vi "Main_VI.vi"() -> ()   [LabVIEW 2023]
uses:
  TypeDef/State.ctl
  TypeDef/Data_Cluster.ctl
  TypeDef/Units.ctl
  TypeDef/Method_Info.ctl
  TypeDef/Method_Types.ctl
panel:
  out "Cluster of Units 2":T1
  out "dmin":dbl format="%#_7g"
  out "dmax":dbl format="%#_7g"
  out "Fundamental Deviation":dbl format="%#_7g"
  out "Cluster of Units":T2
  out "Dmin":dbl format="%#_7g"
  out "Dmax":dbl
  out "Tolerance Grade (IT)":dbl format="%#_7g"
  in  "Help Button":bool
  in  "Close Button":bool
  in  "Base Size":dbl
  in  "Units":T3
  out "Method_Description":string
  out "Symbol":string
  in  "Method_Fit":T4
  in  "error in":errorcluster
  # "Shaft"
  # "Hole"
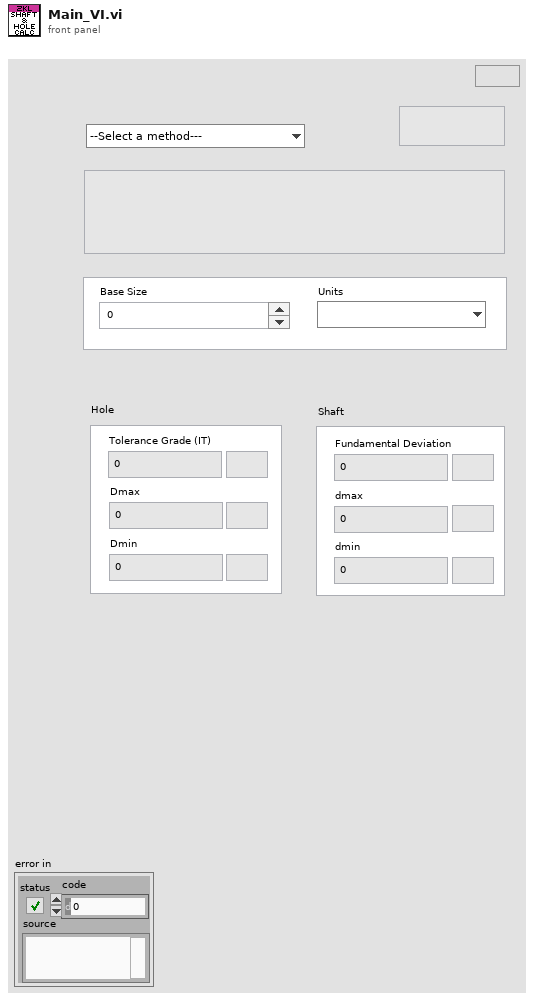
[diagram p1: front panel]
types:
  T1 = cluster{"Units_FundamentalDev":string, "Units_dmax":string, "Units_dmin":string}
  T2 = cluster{"units_it":string, "units_Dmax\nUnits_Dmax":string, "Units_Dmin":string}
  T3 = typedef "Units.ctl" = enum16{"", "mm", "in"}
  T4 = typedef "Method_Types.ctl" = enum16{"--Select a method---", "Clearance (Loose Running Fit)", "Clearance (Free Running Fit)", "Clearance (Close Running Fit)", "Clearance (Sliding Fit)", "Clearance (Locational Fit)", "Transition (Locational A)", "Transition (Locational B)", "Interference (Locational Fit)", "Interference (Force Fit)", "Interference (Medium Drive Fit)"}
  T5 = typedef "Method_Info.ctl" = cluster{"Method":string, "Sym":string, "Tolerance Grade Number":i32, "Shaft":i32, "Group":string}
  T6 = typedef "State.ctl" = enum16{"Wait for something", "Method_Description", "Tolerance Grade Hole", "Dmax-min", "Shaft Fudamental", "Shaft Tolerance Grade", "dmax-dmin", "Write Unit", "End"}
  T7 = typedef "Data_Cluster.ctl" = cluster{"Basic Size ":dbl, "Unit":T3, "Data":T5, "Tolerance Grade Hole  ":dbl, "Fundamental":dbl, "Tables Main Path":path, "Tolerance Grade Shaft":dbl}
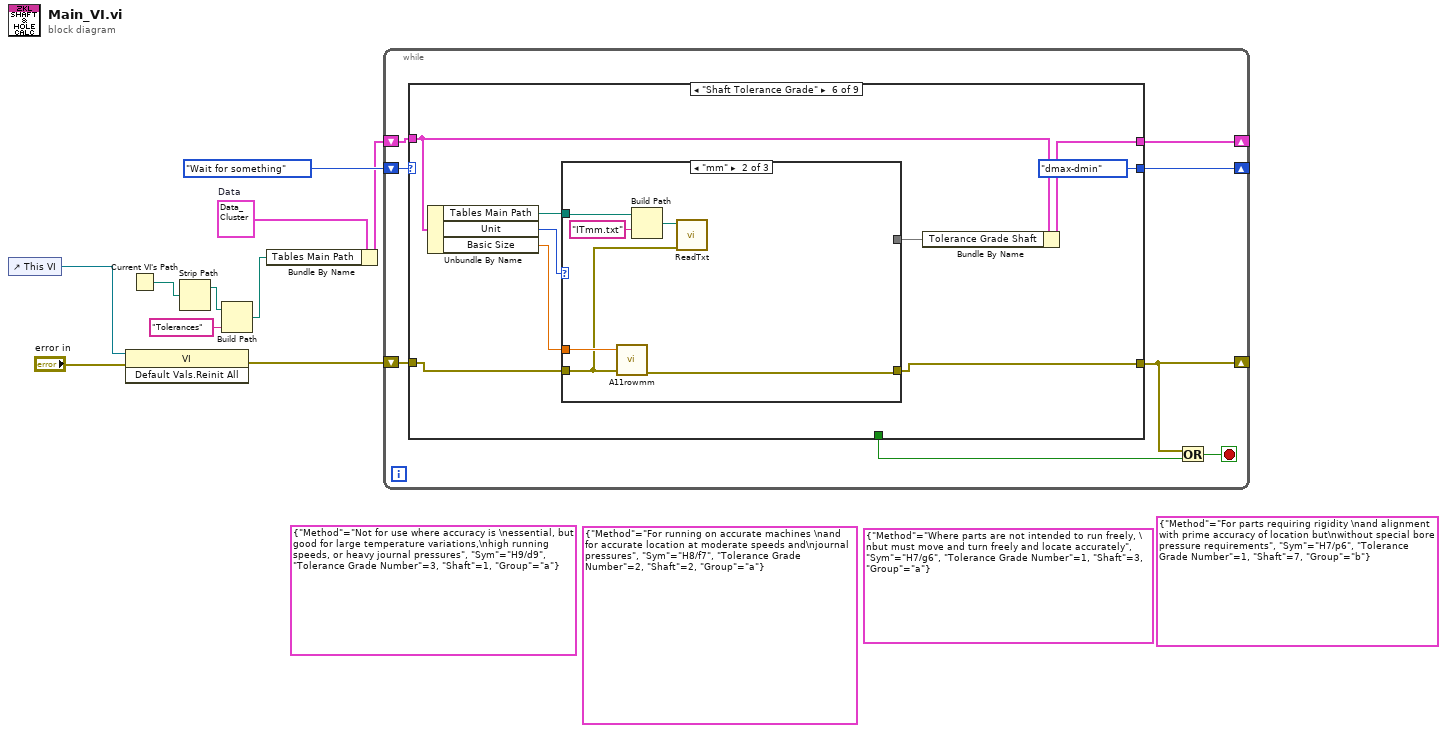
[diagram p0: block diagram]
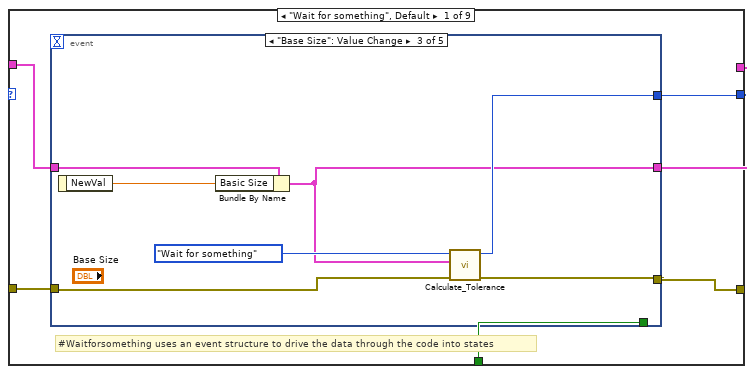
[diagram p2: hidden frame]
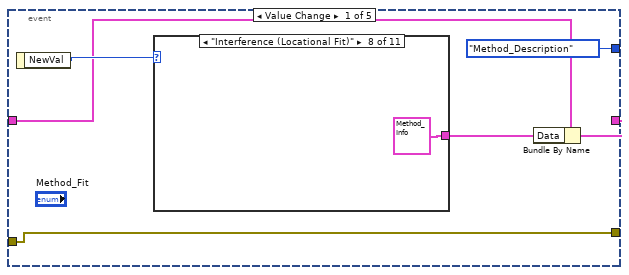
[diagram p3: hidden frame]
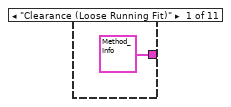
[diagram p4: hidden frame]
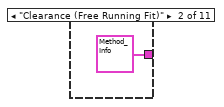
[diagram p5: hidden frame]
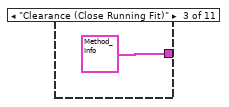
[diagram p6: hidden frame]
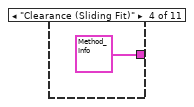
[diagram p7: hidden frame]
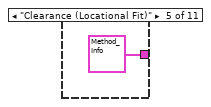
[diagram p8: hidden frame]
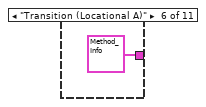
[diagram p9: hidden frame]
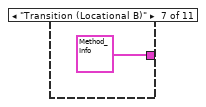
[diagram p10: hidden frame]
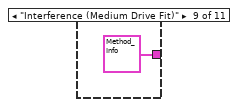
[diagram p11: hidden frame]
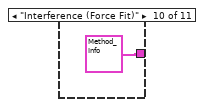
[diagram p12: hidden frame]
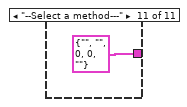
[diagram p13: hidden frame]
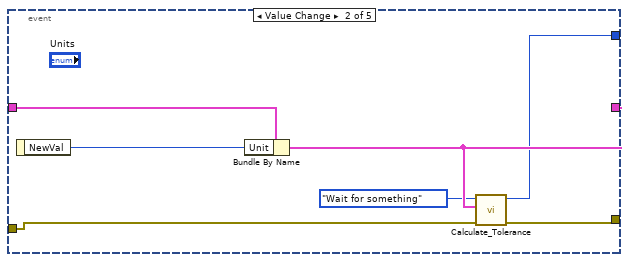
[diagram p14: hidden frame]
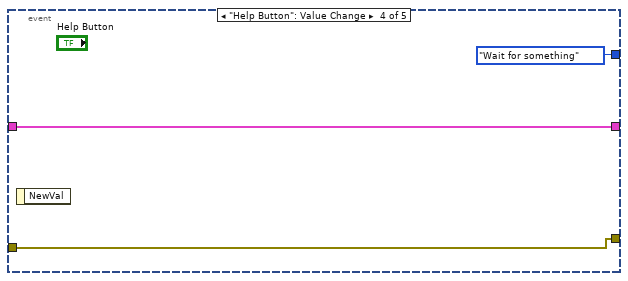
[diagram p15: hidden frame]
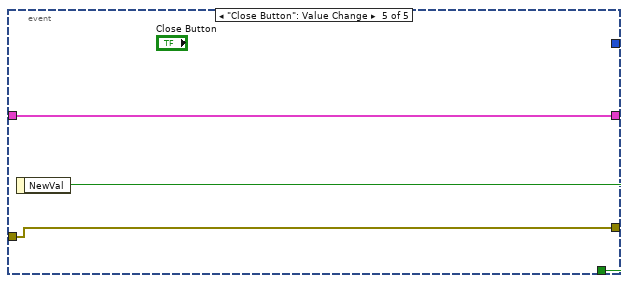
[diagram p16: hidden frame]
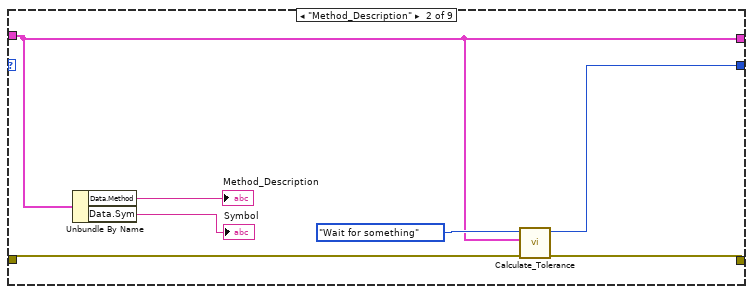
[diagram p17: hidden frame]
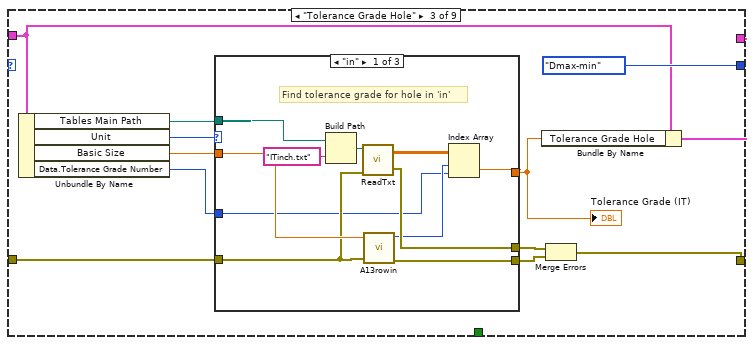
[diagram p18: hidden frame]
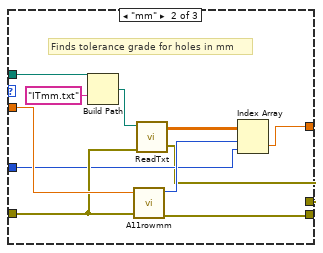
[diagram p19: hidden frame]
diagram:
  (unwired) T5 {"Method"="For parts requiring rigidity \nand alignment with prime accuracy of location but\nwithout special bore pressure requirements", "Sym"="H7/p6", "Tolerance Grade Number"=1, "Shaft"=7, "Group"="b"}
  (unwired) T5 {"Method"="Where parts are not intended to run freely, \nbut must move and turn freely and locate accurately", "Sym"="H7/g6", "Tolerance Grade Number"=1, "Shaft"=3, "Group"="a"}
  (unwired) T5 {"Method"="For running on accurate machines \nand for accurate location at moderate speeds and\njournal pressures", "Sym"="H8/f7", "Tolerance Grade Number"=2, "Shaft"=2, "Group"="a"}
  (unwired) T5 {"Method"="Not for use where accuracy is \nessential, but good for large temperature variations,\nhigh running speeds, or heavy journal pressures", "Sym"="H9/d9", "Tolerance Grade Number"=3, "Shaft"=1, "Group"="a"}
  w10 = T7 {"Basic Size "=0.0, "Unit"=enum."", "Data"={"Method"="", "Sym"="", "Tolerance Grade Number"=0, "Shaft"=0, "Group"=""}, "Tolerance Grade Hole  "=0.0, "Fundamental"=0.0, "Tables Main Path"=path "", "Tolerance Grade Shaft"=0.0}  # Data
  n1 = control-ref of="This VI"() -> (w8:refnum<vi>)
  n2 = invoke class="VI" method="Default Vals.Reinit All"(reference=w8, error in="error in") -> (error out=w6:errorcluster)  [unwired: 1 in, 2 out]
  n3 = Current VI's Path() -> (path=w4:path)
  n4 = Strip Path(path=w4) -> (stripped path=w2:path)  [unwired: 1 out]
  n5 = Build Path(base path=w2, name or relative path="Tolerances") -> (appended path=w3:path)
  n6 = Bundle By Name(cluster=w10, "Tables Main Path"=w3) -> (w5:T7)
  n7 = while {
    shift-right: [w17] -> _
    shift-left: w5 -> [w18]
    shift-right: [w15] -> _
    shift-left: State."Wait for something" -> [w16]
    shift-right: [w11] -> _
    shift-left: w6 -> [w14]
    stop <- w13 stop-if-true
    n8 = case shown="\"Shaft Tolerance Grade\"" w16 {
      tunnel: [w21 w63 w77 w105 w122 w161 w182 w202 w213] -> w17
      tunnel: w18 -> [w24 w63 w76 w105 w131 w163 w182 w202 w213]
      tunnel: [w19 w62 State."Dmax-min" State."Shaft Fudamental" State."Shaft Tolerance Grade" State."dmax-dmin" State."Write Unit" State."Wait for something" State."Wait for something"] -> w15
      tunnel: [w20 w66 w69 w106 w126 w159 w184 w208 w212] -> w11
      tunnel: w14 -> [w23 w65 w79 w107 w128 w160 w184 w209 w212]
      tunnel: [w22 _ _ _ _ _ _ _ _] -> w12
      frame "Wait for something", Default {
        # "#Waitforsomething uses an event structure to drive the data through the code into states"
        n9 = event shown="[2] \"Base Size\": Value Change" {
          selector: _ -> [_ _ _ _ _]
          dyn-events: _ -> [_ _ _ _ _]
          timeout: _ -> [_ _ _ _ _]
          tunnel: [w26 w46 w49 w58 w61] -> w21
          tunnel: w24 -> [w29 w47 w55 w58 w61]
          tunnel: [State."Method_Description" w42 w51 State."Wait for something" _] -> w19
          tunnel: w23 -> [w28 w45 w52 w56 w59]
          tunnel: [_ _ _ _ w60] -> w22
          tunnel: [w28 w43 w53 w56 w59] -> w20
          event Value Change {
            n10 = event-data() -> ("NewVal"=w30:T4)  [unwired: 1 in]
            n11 = case shown="\"Interference (Locational Fit)\"" w30 {
              tunnel: [T5 {"Method"="For wide commercial tolerances or allowances on external members", "Sym"="H11/c11", "Tolerance Grade Number"=5, "Shaft"=0, "Group"="a"} T5 {"Method"="Not for use where accuracy is \nessential, but good for large temperature variations,\nhigh running speeds, or heavy journal pressures", "Sym"="H9/d9", "Tolerance Grade Number"=3, "Shaft"=1, "Group"="a"} T5 {"Method"="For running on accurate machines \nand for accurate location at moderate speeds and\njournal pressures", "Sym"="H8/f7", "Tolerance Grade Number"=2, "Shaft"=2, "Group"="a"} T5 {"Method"="Where parts are not intended to run freely, \nbut must move and turn freely and locate accurately", "Sym"="H7/g6", "Tolerance Grade Number"=1, "Shaft"=3, "Group"="a"} T5 {"Method"="Provides snug fit for location \nof stationary parts, but can be freely assembled and\ndisassembled", "Sym"="H7/h6", "Tolerance Grade Number"=1, "Shaft"=4, "Group"="a"} T5 {"Method"="For accurate location, a \ncompromise between clearance and interference", "Sym"="H7/k6", "Tolerance Grade Number"=1, "Shaft"=5, "Group"="b"} T5 {"Method"="For more accurate location \nwhere greater interference is permissible", "Sym"="H7/n6", "Tolerance Grade Number"=1, "Shaft"=6, "Group"="b"} T5 {"Method"="For parts requiring rigidity \nand alignment with prime accuracy of location but\nwithout special bore pressure requirements", "Sym"="H7/p6", "Tolerance Grade Number"=1, "Shaft"=7, "Group"="b"} T5 {"Method"="For ordinary steel parts or shrink fits on\nlight sections, the tightest fit usable with cast iron", "Sym"="H7/s6", "Tolerance Grade Number"=1, "Shaft"=8, "Group"="b"} T5 {"Method"="Suitable for parts that can be highly stressed \nor for shrink fits where the heavy pressing forces required\nare impractical", "Sym"="H7/u6", "Tolerance Grade Number"=1, "Shaft"=9, "Group"="b"} T5 {"Method"="", "Sym"="", "Tolerance Grade Number"=0, "Shaft"=0, "Group"=""}] -> w25
              frame "Clearance (Loose Running Fit)" {
              }
              frame "Clearance (Free Running Fit)" {
              }
              frame "Clearance (Close Running Fit)" {
              }
              frame "Clearance (Sliding Fit)" {
              }
              frame "Clearance (Locational Fit)" {
              }
              frame "Transition (Locational A)" {
              }
              frame "Transition (Locational B)" {
              }
              frame "Interference (Locational Fit)" {
              }
              frame "Interference (Medium Drive Fit)" {
              }
              frame "Interference (Force Fit)" {
              }
              frame "--Select a method---" {
              }
            }
            n12 = Bundle By Name(cluster=w29, "Data"=w25) -> (w26:T7)
          }
          event Value Change {
            n13 = event-data() -> ("NewVal"=w48:T3)  [unwired: 1 in]
            n14 = Bundle By Name(cluster=w47, "Unit"=w48) -> (w46:T7)
            n15 = call "Calculate_Tolerance.vi"("error in (no error)"=w45, "Data"=w46, "State"=State."Wait for something") -> ("error out"=w43:errorcluster, "State"=w42:T6)  [unwired: 7 in]
          }
          event "Base Size": Value Change {
            n16 = event-data() -> ("NewVal"=w54:dbl)  [unwired: 1 in]
            n17 = Bundle By Name(cluster=w55, "Basic Size"=w54) -> (w49:T7)
            n18 = call "Calculate_Tolerance.vi"("error in (no error)"=w52, "Data"=w49, "State"=State."Wait for something") -> ("error out"=w53:errorcluster, "State"=w51:T6)  [unwired: 7 in]
          }
          event "Help Button": Value Change {
            n19 = event-data() -> ()  [unwired: 1 in, 1 out]
          }
          event "Close Button": Value Change {
            n20 = event-data() -> ("NewVal"=w60:bool)  [unwired: 1 in]
          }
        }
      }
      frame "Method_Description" {
        n21 = Unbundle By Name(w63) -> ("Data.Method"=→"Method_Description":string, "Data.Sym"=→"Symbol":string)
        n22 = call "Calculate_Tolerance.vi"("error in (no error)"=w65, "Data"=w63, "State"=State."Wait for something") -> ("error out"=w66:errorcluster, "State"=w62:T6)  [unwired: 7 in]
      }
      frame "Tolerance Grade Hole" {
        n23 = Unbundle By Name(w76) -> ("Tables Main Path"=w73:path, "Unit"=w78:T3, "Basic Size"=w75:dbl, "Data.Tolerance Grade Number"=w72:i32)
        n24 = case shown="\"in\"" w78 {
          tunnel: w79 -> [w89 w101 w103]
          tunnel: [w81 w94 _] -> w74
          tunnel: w75 -> [w90 w102 _]
          tunnel: w73 -> [w88 w100 _]
          tunnel: w72 -> [w82 w95 _]
          tunnel: [w85 w93 w103] -> w71
          tunnel: [w84 w92 _] -> w70
          frame "in" {
            # "Find tolerance grade for hole in 'in'"
            n25 = Build Path(base path=w88, name or relative path="ITinch.txt") -> (appended path=w87:path)
            n26 = call "ReadTxt.vi"("error in"=w89, "ITmm path"=w87) -> ("error out"=w85:errorcluster, "Table IT Grade"=w91:ext[][])  [unwired: 4 in]
            n27 = call "A13rowin.vi"("Basic Size"=w90, "error in"=w89) -> ("Row"=w83:i32, "error out"=w84:errorcluster)  [unwired: 5 in]
            n28 = Index Array(array=w91, index (row)=w83, index (col)=w82) -> (element=w81:ext)
          }
          frame "mm" {
            # "Finds tolerance grade for holes in mm"
            n29 = Build Path(base path=w100, name or relative path="ITmm.txt") -> (appended path=w99:path)
            n30 = call "A11rowmm.vi"("Basic Size"=w102, "error in (no error)"=w101) -> ("Row"=w97:i32, "error out"=w92:errorcluster)  [unwired: 5 in]
            n31 = call "ReadTxt.vi"("error in"=w101, "ITmm path"=w99) -> ("error out"=w93:errorcluster, "Table IT Grade"=w96:ext[][])  [unwired: 4 in]
            n32 = Index Array(array=w96, index (row)=w97, index (col)=w95) -> (element=w94:ext)
          }
          frame "" {
          }
        }
        "Tolerance Grade (IT)" <- w74
        n33 = Bundle By Name(cluster=w76, "Tolerance Grade Hole"=w74) -> (w77:T7)
        n34 = Merge Errors(w71, w70) -> (w69:errorcluster)
      }
      frame "Dmax-min" {
        n35 = Unbundle By Name(w105) -> ("Tolerance Grade Hole"=w104:dbl, "Basic Size"=w111:dbl, "Unit"=w110:T3)
        n36 = case shown="\"mm\"" w110 {
          tunnel: w104 -> [w115 w119]
          tunnel: w111 -> [w114 w118]
          tunnel: [w116 w120] -> w109
          tunnel: [w114 w118] -> w108
          tunnel: w107 -> [w113 w117]
          tunnel: [w113 w117] -> w106
          frame "in", Default {
            # "inch"
            n37 = Add(x=w115, y=w114) -> (x+y=w116:dbl)
          }
          frame "mm" {
            # "in mm"
            n38 = Add(x=w119, y=w118) -> (x+y=w120:dbl)
          }
        }
        "Dmax" <- w109
        "Dmin" <- w108
      }
      frame "Shaft Fudamental" {
        n39 = Unbundle By Name(w131) -> ("Tables Main Path"=w124:path, "Unit"=w129:T3, "Data.Shaft"=w130:i32, "Basic Size"=w123:dbl)
        n40 = case shown="\"mm\"" w129 {
          tunnel: w130 -> [w134 w145 _]
          tunnel: w123 -> [w142 w153 _]
          tunnel: [w133 w144 _] -> w121
          tunnel: w128 -> [w141 w151 w155]
          tunnel: [w139 w152 w155] -> w127
          tunnel: [w140 w150 _] -> w125
          tunnel: w124 -> [w137 w147 _]
          frame "in", Default {
            # "Shaft inches"
            n41 = call "A14rowin.vi"("Basic Size"=w142, "error in (no error)"=w141) -> ("Row"=w135:i32, "error out"=w140:errorcluster)  [unwired: 5 in]
            n42 = Build Path(base path=w137, name or relative path="ShaftIn.txt") -> (appended path=w136:path)
            n43 = call "ReadTxt.vi"("error in"=w141, "ITmm path"=w136) -> ("error out"=w139:errorcluster, "Table IT Grade"=w143:ext[][])  [unwired: 4 in]
            n44 = Index Array(array=w143, index (row)=w135, index (col)=w134) -> (element=w133:ext)
          }
          frame "mm" {
            # "Shaft fundamental dev in mm"
            n45 = call "Find_Row_Shaft-mm.vi"("Basic Size"=w153, "error in"=w151) -> ("Row"=w146:i32, "error out"=w150:errorcluster)  [unwired: 5 in]
            n46 = Build Path(base path=w147, name or relative path="Shaftmm.txt") -> (appended path=w148:path)
            n47 = call "ReadTxt.vi"("error in"=w151, "ITmm path"=w148) -> ("error out"=w152:errorcluster, "Table IT Grade"=w154:ext[][])  [unwired: 4 in]
            n48 = Index Array(array=w154, index (row)=w146, index (col)=w145) -> (element=w144:ext)
          }
          frame "" {
          }
        }
        "Fundamental Deviation" <- w121
        n49 = Bundle By Name(cluster=w131, "Fundamental"=w121) -> (w122:T7)
        n50 = Merge Errors(w127, w125) -> (w126:errorcluster)
      }
      frame "Shaft Tolerance Grade" {
        n51 = Unbundle By Name(w163) -> ("Tables Main Path"=w158:path, "Unit"=w162:T3, "Basic Size"=w157:dbl)
        n52 = case shown="\"mm\"" w162 {
          tunnel: w160 -> [w165 w166 w172]
          tunnel: [w165 w168 w174] -> w159
          tunnel: w158 -> [_ w169 w175]
          tunnel: w157 -> [_ w167 w173]
          tunnel: [_ _ _] -> w156
          frame "", Default {
          }
          frame "mm" {
            n53 = call "A11rowmm.vi"("Basic Size"=w167, "error in (no error)"=w166) -> ("error out"=w168:errorcluster)  [unwired: 5 in, 1 out]
            n54 = Build Path(base path=w169, name or relative path="ITmm.txt") -> (appended path=w171:path)
            n55 = call "ReadTxt.vi"("error in"=w166, "ITmm path"=w171) -> ()  [unwired: 4 in, 2 out]
          }
          frame "in" {
            n56 = call "A13rowin.vi"("Basic Size"=w173, "error in"=w172) -> ("error out"=w174:errorcluster)  [unwired: 5 in, 1 out]
            n57 = Build Path(base path=w175, name or relative path="ITinch.txt") -> (appended path=w177:path)
            n58 = call "ReadTxt.vi"("error in"=w172, "ITmm path"=w177) -> ()  [unwired: 4 in, 2 out]
          }
        }
        n59 = Bundle By Name(cluster=w163, "Tolerance Grade Shaft"=w156) -> (w161:T7)
      }
      frame "dmax-dmin" {
        n60 = Unbundle By Name(w182) -> ("Data.Group"=w180:string, "Basic Size"=w186:dbl, "Fundamental"=w185:dbl, "Tolerance Grade Shaft"=w183:dbl, "Unit"=w181:T3)
        n61 = case shown="\"mm\"" w181 {
          tunnel: w186 -> [_ w190 _]
          tunnel: w185 -> [_ w189 _]
          tunnel: w183 -> [_ w188 _]
          tunnel: w180 -> [_ w193 w201]
          tunnel: [_ w192 _] -> w179
          tunnel: [_ w191 _] -> w178
          frame "", Default {
          }
          frame "mm" {
            n62 = case shown="\"a\"" w193 {
              tunnel: [_ w198] -> w192
              tunnel: [w194 w199] -> w191
              tunnel: w190 -> [w196 w200]
              tunnel: w189 -> [w195 w197]
              tunnel: w188 -> [_ _]
              frame "b", Default {
                n63 = Add(x=w196, y=w195) -> (x+y=w194:dbl)
              }
              frame "a" {
                n64 = Add(x=w200, y=w197) -> (x+y=w198:dbl)
                n65 = Subtract(x=w198) -> (x-y=w199:dbl)  [unwired: 1 in]
              }
            }
          }
          frame "in" {
            n66 = case shown="\"b\", Default" w201 {
              frame "b", Default {
              }
              frame "a" {
              }
            }
          }
        }
        "dmax" <- w179
        "dmin" <- w178
      }
      frame "Write Unit" {
        # "I used clusters just because I liked the esthetics, could have been an array\nor making the paramters strings and concatenate with the unit at the end"
        n67 = Unbundle By Name(w202) -> ("Unit"=w210:T3)
        n68 = Format Into String(error in=w209, w210) -> (resulting string=w203:string, error out=w208:errorcluster)  [unwired: 2 in]
        n69 = Bundle By Name(cluster=T2 {"units_it"="", "units_Dmax\nUnits_Dmax"="", "Units_Dmin"=""} ("Cluster of Units"), "units_it"=w203, "units_Dmax\nUnits_Dmax"=w203, "Units_Dmin"=w203) -> (→"Cluster of Units":T2)
        n70 = Bundle By Name(cluster=T1 {"Units_FundamentalDev"="", "Units_dmax"="", "Units_dmin"=""} ("Cluster of Units 2"), "Units_FundamentalDev"=w203, "Units_dmax"=w203, "Units_dmin"=w203) -> (→"Cluster of Units 2":T1)
      }
      frame "End" {
      }
    }
    n71 = Or(x=w11, y=w12) -> (x .or. y?=w13:bool)
  }
